vi "LVFunction_Get installed HASO sensor list from selected folder.vi"(0 "FolderToScan":path) -> (4 "Array_Of_HASO_specifications":T5(array[cluster]), 6 "ArrayOfConfigFilePath":path[](array[path]), 8 "Installed sensors":string[](array[string]), 10 "HasoModelList":string[](array[string]))   [LabVIEW 2020]
uses:
  HasoSpecifications.ctl
  General dimensions definition.ctl
  Point2D.ctl
  Point2Df.ctl
  Remove Duplicates from 1D Array (String)__ogtk.vi
panel:
  in  "String 2":string
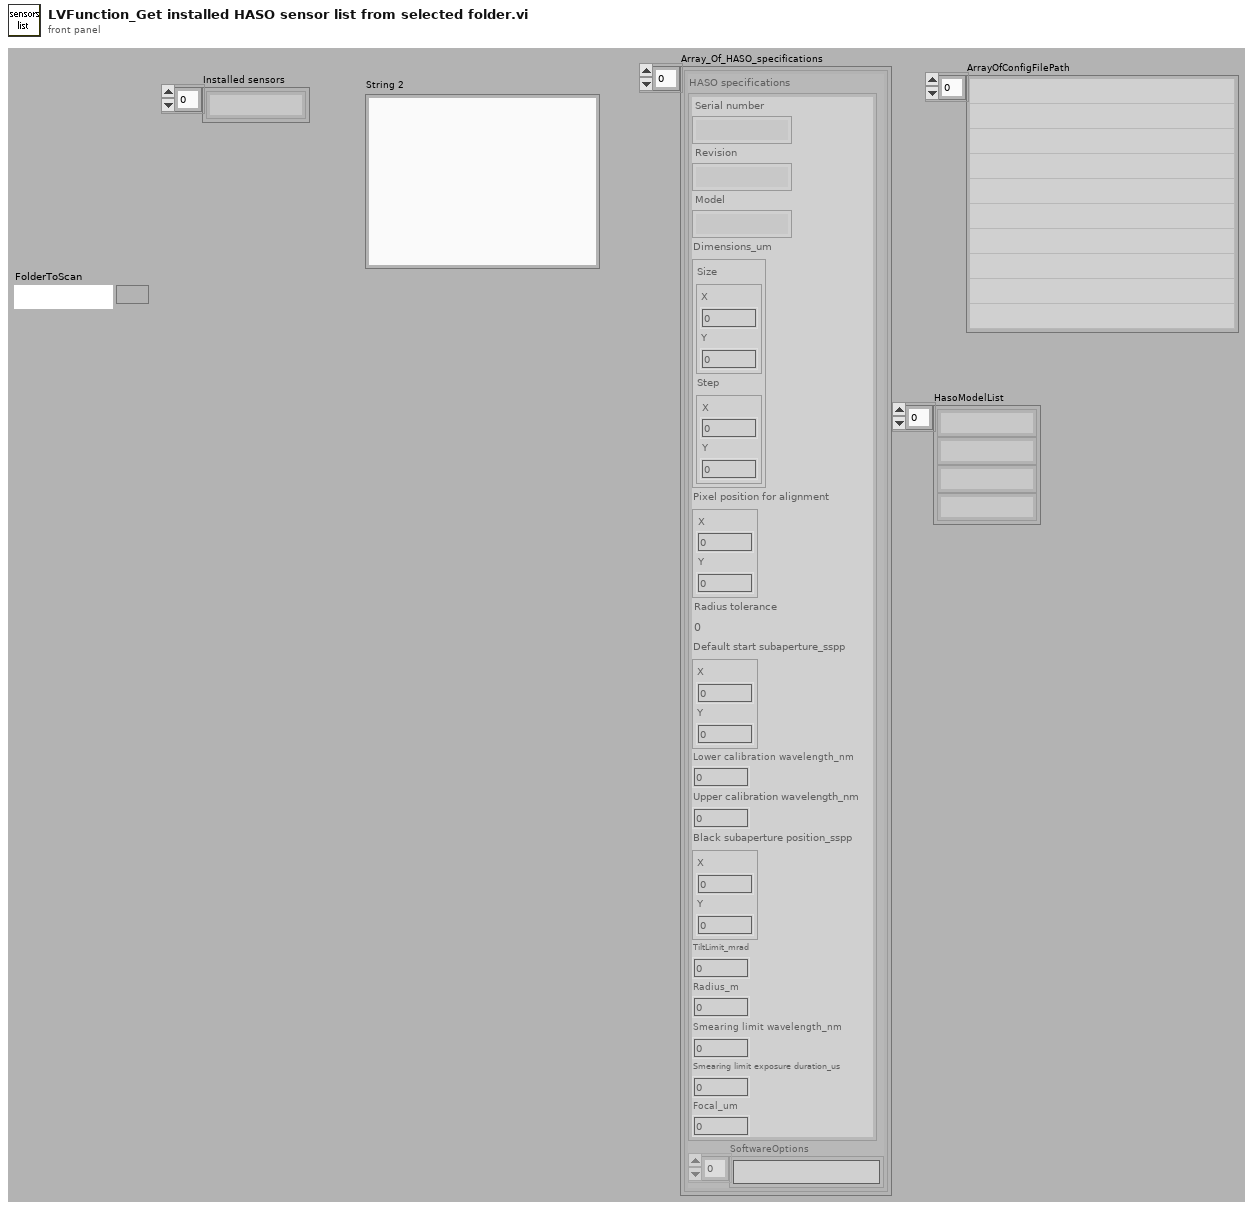
[diagram p1: front panel]
types:
  T1 = typedef "HasoSpecifications.ctl" = cluster{"Serial number":string, "Revision":string, "Model":string, "Dimensions_um":T2, "Pixel position for alignment":T4, "Radius tolerance":u16, "Default start subaperture_sspp":T3, "Lower calibration wavelength_nm":dbl, "Upper calibration wavelength_nm":dbl, "Black subaperture position_sspp":T3, "TiltLimit_mrad":dbl, "Radius_m":dbl, "Smearing limit wavelength_nm":dbl, "Smearing limit exposure duration_us":dbl, "Focal_um":dbl}
  T2 = typedef "General dimensions definition.ctl" = cluster{"Size":T3, "Step":T4}
  T3 = typedef "Point2D.ctl" = cluster{"X":u32, "Y":u32}
  T4 = typedef "Point2Df.ctl" = cluster{"X":sgl, "Y":sgl}
  T5 = cluster{"HASO specifications":T1, "SoftwareOptions":string[]}[]
  T6 = cluster{"HASO specifications":T1, "SoftwareOptionsList":string[]}
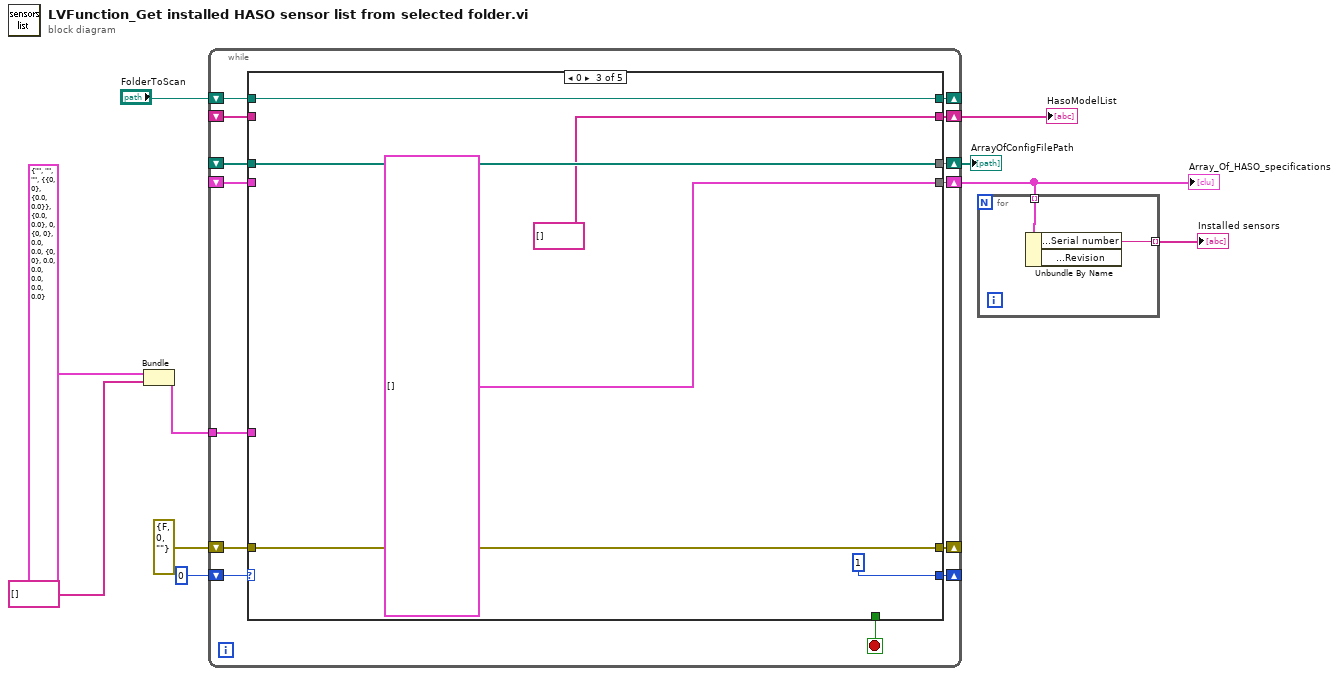
[diagram p0: block diagram]
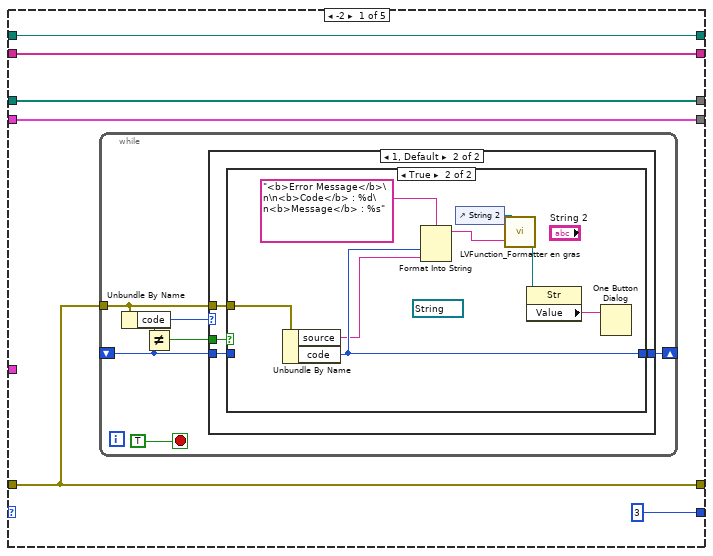
[diagram p2: hidden frame]
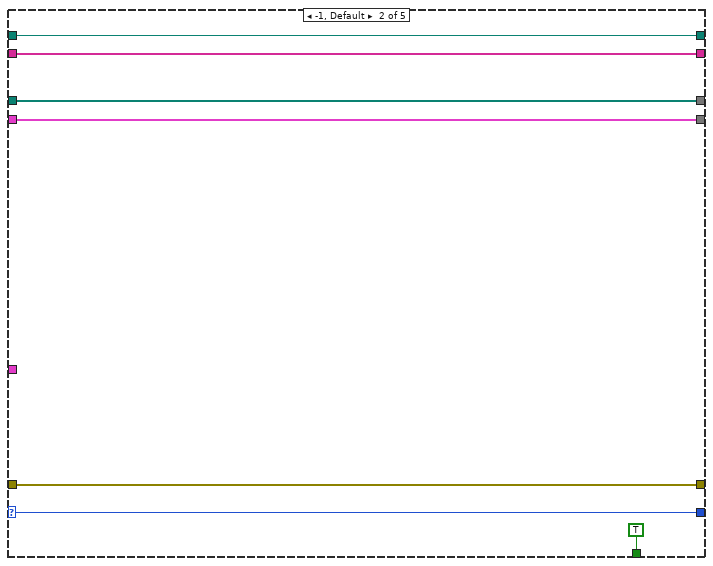
[diagram p5: hidden frame]
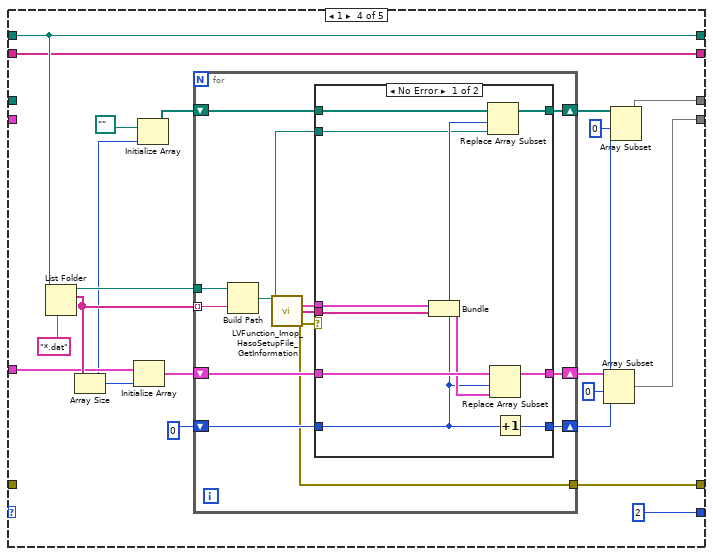
[diagram p6: hidden frame]
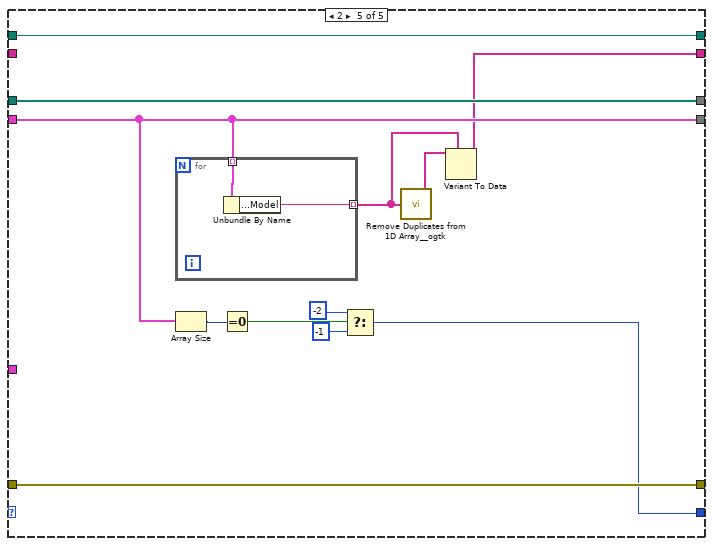
[diagram p8: hidden frame]
diagram:
  n1 = Bundle("HASO specifications"=T1 {"Serial number"="", "Revision"="", "Model"="", "Dimensions_um"={"Size"={"X"=0, "Y"=0}, "Step"={"X"=0.0, "Y"=0.0}}, "Pixel position for alignment"={"X"=0.0, "Y"=0.0}, "Radius tolerance"=0, "Default start subaperture_sspp"={"X"=0, "Y"=0}, "Lower calibration wavelength_nm"=0.0, "Upper calibration wavelength_nm"=0.0, "Black subaperture position_sspp"={"X"=0, "Y"=0}, "TiltLimit_mrad"=0.0, "Radius_m"=0.0, "Smearing limit wavelength_nm"=0.0, "Smearing limit exposure duration_us"=0.0, "Focal_um"=0.0}, string[] []) -> (w7:cluster{"HASO specifications":T1, string[]})  [unwired: 1 in]
  n2 = while {
    shift-right: [w19] -> _
    shift-left: 0 -> [w24]
    shift-right: [w22] -> w5
    shift-left: _ -> [w21]
    tunnel: w7 -> [w23]
    shift-right: [w17] -> _
    shift-left: errorcluster {"status"=FALSE, "code"=0, "source"=""} ("error out") -> [w18]
    shift-right: [w16] -> w3
    shift-left: _ -> [w15]
    shift-right: [w14] -> _
    shift-left: "FolderToScan" -> [w13]
    shift-right: [w12] -> w2
    shift-left: _ -> [w11]
    stop <- w20 stop-if-true
    n3 = case shown="0" w24 {
      selector: w24 -> [_ w55 _ _ _]
      tunnel: w23 -> [_ _ _ w80 _]
      tunnel: [w28 w57 cluster{"HASO specifications":T1, string[]}[] [] w76 w110] -> w22
      tunnel: w21 -> [w28 w57 _ _ w110]
      tunnel: [_ TRUE _ _ _] -> w20
      tunnel: [3 w55 1 2 w115] -> w19
      tunnel: w18 -> [w30 w54 w63 _ w120]
      tunnel: [w30 w54 w63 w73 w120] -> w17
      tunnel: [w27 w53 w62 w68 w119] -> w16
      tunnel: w15 -> [w27 w53 w62 _ w119]
      tunnel: [w26 w52 w58 w66 w118] -> w14
      tunnel: w13 -> [w26 w52 w58 w66 w118]
      tunnel: [w25 w51 string[] [] w64 w109] -> w12
      tunnel: w11 -> [w25 w51 _ w64 _]
      frame -2 {
        n4 = while {
          tunnel: w30 -> [w36]
          shift-right: [w35] -> _
          shift-left: _ -> [w34]
          stop <- TRUE stop-if-true
          n5 = Unbundle By Name(w36) -> ("code"=w31:i32)
          n6 = Not Equal?(x=w31, y=w34) -> (x != y?=w32:bool)
          n7 = case shown="1, Default" w31 {
            selector: w31 -> [w37 _]
            tunnel: w36 -> [_ w41]
            tunnel: [w37 w40] -> w35
            tunnel: w34 -> [_ w39]
            tunnel: w32 -> [_ w38]
            frame 0 {
            }
            frame 1, Default {
              n8 = case shown="True" w38 {
                tunnel: w41 -> [_ w50]
                tunnel: [w42 w49] -> w40
                tunnel: w39 -> [w42 _]
                frame False {
                }
                frame True {
                  (unwired) refnum<vi> refnum ("String to Format (not a refnum)")
                  n9 = Unbundle By Name(w50) -> ("source"=w48:string, "code"=w49:i32)
                  n10 = Format Into String(format string="<b>Error Message</b>\n\n<b>Code</b> : %d\n<b>Message</b> : %s" ("initial string"), w49, w48) -> (resulting string=w44:string)  [unwired: 2 in, 1 out]
                  n11 = control-ref of="String 2"() -> (w45:refnum<vi>)
                  n12 = call "LVFunction_Formatter en gras.vi"("Chaîne"=w44, "Contrôle chaîne"=w45) -> ("Contrôle chaîne (dup)"=w43:refnum<vi>)  [unwired: 1 in]
                  n13 = property class="Str"(reference=w43) -> ("Value"=w46:string)  [unwired: 1 in, 2 out]
                  n14 = One Button Dialog(message=w46) -> ()  [unwired: 1 in, 1 out]
                }
              }
            }
          }
        }
      }
      frame -1, Default {
      }
      frame 0 {
      }
      frame 1 {
        n15 = List Folder(path=w66, pattern="*.dat") -> (path out=w82:path, filenames=w81:string[])  [unwired: 2 in, 2 out]
        n16 = Array Size(array=w81) -> (size(s)=w72:i32)
        n17 = Initialize Array(w80, w72) -> (w79:cluster{"HASO specifications":T1, string[]}[])
        n18 = Initialize Array(path "" ("appended path"), w72) -> (w67:path[])
        n19 = for {
          tunnel: w82 -> [w95]
          tunnel: w81 -> [w94] mode=indexing
          shift-right: [w91] -> w77
          shift-left: w79 -> [w93]
          shift-right: [w88] -> w65
          shift-left: 0 -> [w92]
          tunnel: [w87] -> w73
          shift-right: [w85] -> w69
          shift-left: w67 -> [w86]
          n20 = Build Path(base path=w95, name or relative path=w94) -> (appended path=w84:path)
          n21 = call "LVFunction_Imop_HasoSetupFile_GetInformation.vi"("WFS_setup_file IN"=w84) -> ("HASO specifications"=w90:T1, "SoftwareOptionsList"=w89:string[], "error out"=w87:errorcluster)  [unwired: 10 in, 2 out]
          n22 = case shown="No Error" w87 {
            tunnel: w93 -> [w105 w108]
            tunnel: w92 -> [w99 w107]
            tunnel: [w104 w108] -> w91
            tunnel: w90 -> [w97 _]
            tunnel: w89 -> [w96 _]
            tunnel: [w102 w107] -> w88
            tunnel: w86 -> [w101 w106]
            tunnel: [w100 w106] -> w85
            tunnel: w84 -> [w98 _]
            frame No Error {
              n23 = Bundle("HASO specifications"=w97, "SoftwareOptionsList"=w96) -> (w103:T6)  [unwired: 1 in]
              n24 = Replace Array Subset(array=w101, new element=w98, index=w99) -> (w100:path[])
              n25 = Replace Array Subset(array=w105, new element=w103, index=w99) -> (w104:cluster{"HASO specifications":T1, string[]}[])
              n26 = Increment(x=w99) -> (x+1=w102:i32)
            }
            frame Error {
            }
          }
        }
        n27 = Array Subset(array=w77, index=0, length=w65) -> (w76:cluster{"HASO specifications":T1, string[]}[])
        n28 = Array Subset(array=w69, index=0, length=w65) -> (w68:path[])
      }
      frame 2 {
        n29 = for {
          tunnel: w110 -> [w122] mode=indexing
          tunnel: [w121] -> w111 mode=indexing
          n30 = Unbundle By Name(w122) -> ("HASO specifications.Model"=w121:string)
        }
        n31 = Array Size(array=w110) -> (size(s)=w117:i32)
        n32 = Equal To 0?(x=w117) -> (x = 0?=w116:bool)
        n33 = Select(t=-2, s=w116, f=-1) -> (s? t:f=w115:i32)
        n34 = call-poly "Remove Duplicates from 1D Array__ogtk.vi"("Input Array"=w111) -> ("Output Array"=w112:string[])  [unwired: 1 out]
        n35 = Variant To Data(type=w111, Variant=w112) -> (data=w109:string[])  [unwired: 1 in, 1 out]
      }
    }
  }
  "Array_Of_HASO_specifications" <- w5
  "ArrayOfConfigFilePath" <- w3
  "HasoModelList" <- w2
  n36 = for {
    tunnel: w5 -> [w124] mode=indexing
    tunnel: [w123] -> w4 mode=indexing
    n37 = Unbundle By Name(w124) -> ("HASO specifications.Serial number"=w123:string)  [unwired: 1 out]
  }
  "Installed sensors" <- w4
